vi "3DObjectManipulation.vi"() -> ()   [LabVIEW 2011]
uses:
  <vilib>/picture/3D Picture Control/NI_3D Picture Control.lvlib
panel:
  in  "stop":bool
  out "3D Picture":refnum<vi>(3d-picture)
  in  "Translation":cluster{"X":sgl, "Y":sgl, "Z":sgl}
  in  "Scale":cluster{"X":sgl, "Y":sgl, "Z":sgl}={"X"=1.457233, "Y"=1.0, "Z"=1.0} {"X" scale=0.0..5.0; "Y" scale=0.0..5.0; "Z" scale=0.0..5.0}
  out "Axis 2":cluster{"X":sgl, "Y":sgl, "Z":sgl}={"X"=0.70710677, "Y"=0.70710677, "Z"=0.0}
  in  "Angle":sgl=15.0
  in  "Axis":cluster{"X":sgl, "Y":sgl, "Z":sgl}={"X"=0.0, "Y"=1.0, "Z"=0.0}
  in  "Color":T1={"Red"=0.21212122, "Green"=1.0, "Blue"=0.54545456, "Alpha"=1.0} {"Red" scale=0.0..1.0; "Green" scale=0.0..1.0; "Blue" scale=0.0..1.0}
  in  "Length Z":sgl=1.0
  in  "Length X":sgl=1.0
  in  "Length Y":sgl=1.0
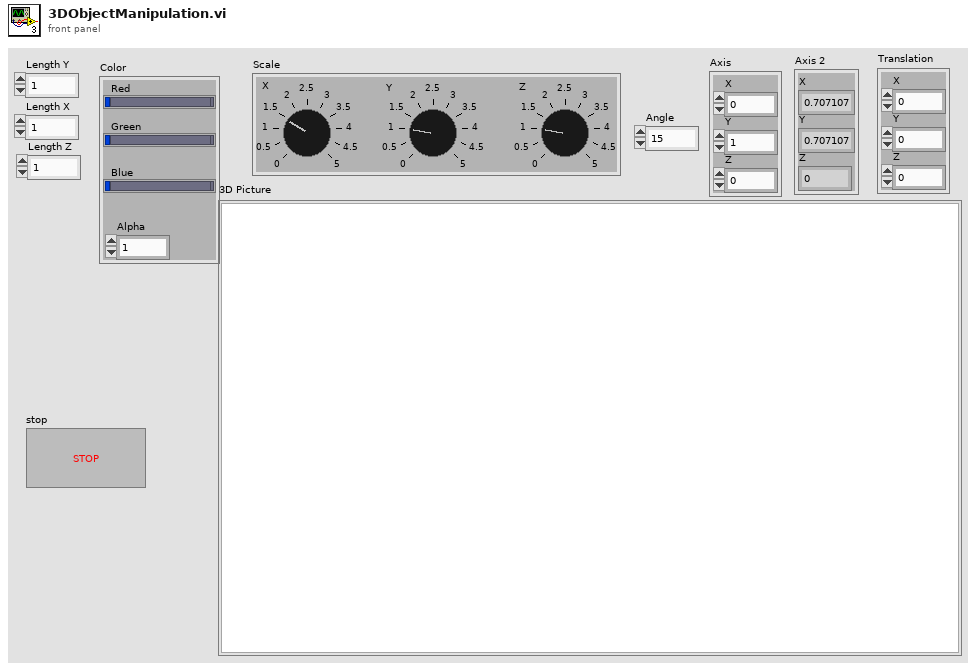
[diagram p1: front panel]
types:
  T1 = cluster{"Red":sgl, "Green":sgl, "Blue":sgl, "Alpha":sgl}
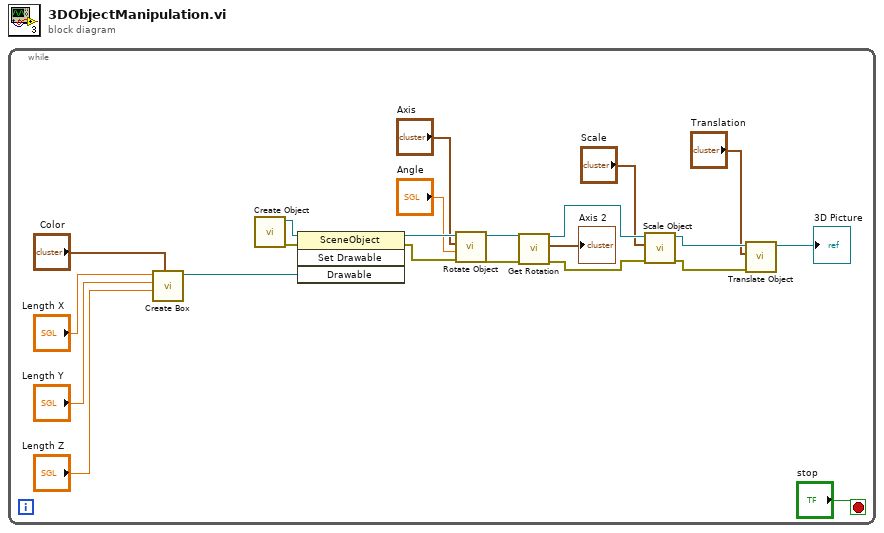
[diagram p0: block diagram]
diagram:
  n1 = while {
    stop <- "stop" stop-if-true
    n2 = call <vilib>:"Create Box.vi"("Color"="Color", "Length Z"="Length Z", "Length Y"="Length Y", "Length X"="Length X") -> ("New Box Refnum"=w20:refnum<vi>)  [unwired: 6 in, 1 out]
    n3 = call <vilib>:"Create Object.vi"() -> ("error out"=w21:errorcluster, "Scene:New Object"=w22:refnum<vi>)  [unwired: 10 in]
    n4 = invoke class="SceneObject" method="Set Drawable"(reference=w22, error in=w21, "Drawable"=w20) -> (reference out=w15:refnum<vi>, error out=w14:errorcluster)  [unwired: 1 in, 2 out]
    n5 = call <vilib>:"Rotate Object.vi"("error in (no error)"=w14, "Angle"="Angle", "Axis"="Axis", "Scene.Object In"=w15) -> ("error out"=w10:errorcluster, "Scene.Object Out"=w11:refnum<vi>)  [unwired: 6 in]
    n6 = call <vilib>:"Get Rotation.vi"("error in (no error)"=w10, "Scene Object"=w11) -> ("error out"=w7:errorcluster, "Axis"=→"Axis 2":cluster{"X":sgl, "Y":sgl, "Z":sgl}, "Scene Object"=w8:refnum<vi>)  [unwired: 6 in, 1 out]
    n7 = call <vilib>:"Scale Object.vi"("error in (no error)"=w7, "Scale"="Scale", "Scene.Object In"=w8) -> ("error out"=w4:errorcluster, "Scene.Object Out"=w5:refnum<vi>)  [unwired: 7 in]
    n8 = call <vilib>:"Translate Object.vi"("error in (no error)"=w4, "Translation"="Translation", "Scene.Object In"=w5) -> ("Scene.Object Out"=→"3D Picture":refnum<vi>)  [unwired: 7 in, 1 out]
  }
